vi "Config.vi"(8 "error in (no error)":errorcluster, 10 "Setting":variant, 11 "APS 7050":refnum<class "APS 7050.lvclass">) -> (0 "error out":errorcluster, 3 "APS 7050 out":refnum<class "APS 7050.lvclass">)   [LabVIEW 2025, in "Power Supply.lvlib" / "APS 7050.lvclass"]
uses:
  APS 7050.lvclass
  APS 7050.lvclass/APS 7050.ctl
  <instrlib>/APS-7000 Series/APS-7000 Series.lvlib
  PS Channel/Power Supply Channel.lvclass
  PS Channel configuration/Power Supply Channel configuration.lvclass
  Users/Public/Documents/Sandia National Labs/TSS Plugin/Abstract Engine.lvlibp/Plugin/Abstract/Abstract Instrument/Channel.ctl
  Users/Public/Documents/Sandia National Labs/TSS Plugin/Abstract Engine.lvlibp/Plugin/Abstract/Abstract Instrument/Abstract Instrument.lvclass
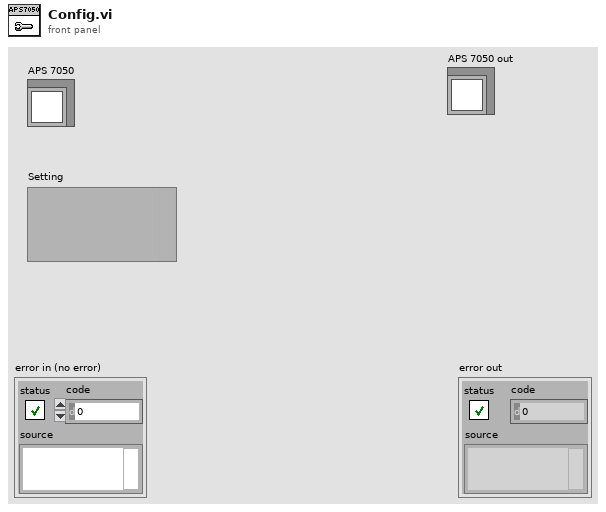
[diagram p1: front panel]
types:
  T1 = typedef "Abstract Engine.lvlibp/Abstract Instrument.lvclass/Channel.ctl" = cluster{"Alias":string, "DataType":enum16{"Anaolg Input", "Waveform"}, "Unit":enum16{"---", "V", "A", "Ohm", "Hz", "uF", "degC", "deg"}, "Upper limit":dbl, "Lower limit":dbl, "Measurement":variant}
  T2 = cluster{"Range":enum16{"R155", "R310", "R600", "AUTO"}, "FREQ":dbl, "ACV":dbl}
  T3 = typedef "Power Supply.lvlib/Power Supply Channel configuration.lvclass/PS Channel Setting.ctl" = cluster{"Driver":string, "Pin":string, "Test Voltage":string, "Voltage Low":dbl, "Voltage Norminal":dbl, "Voltage High":dbl, "PreTest Voltage":dbl, "PreTest Current":dbl, "Current Limit":dbl}
  T4 = typedef "Abstract Engine.lvlibp/Channel configuration.lvclass/Default Channel.ctl" = cluster{"Address":string, "SW Alias":string, "Enabled":bool, "Type":string, "Description":string}
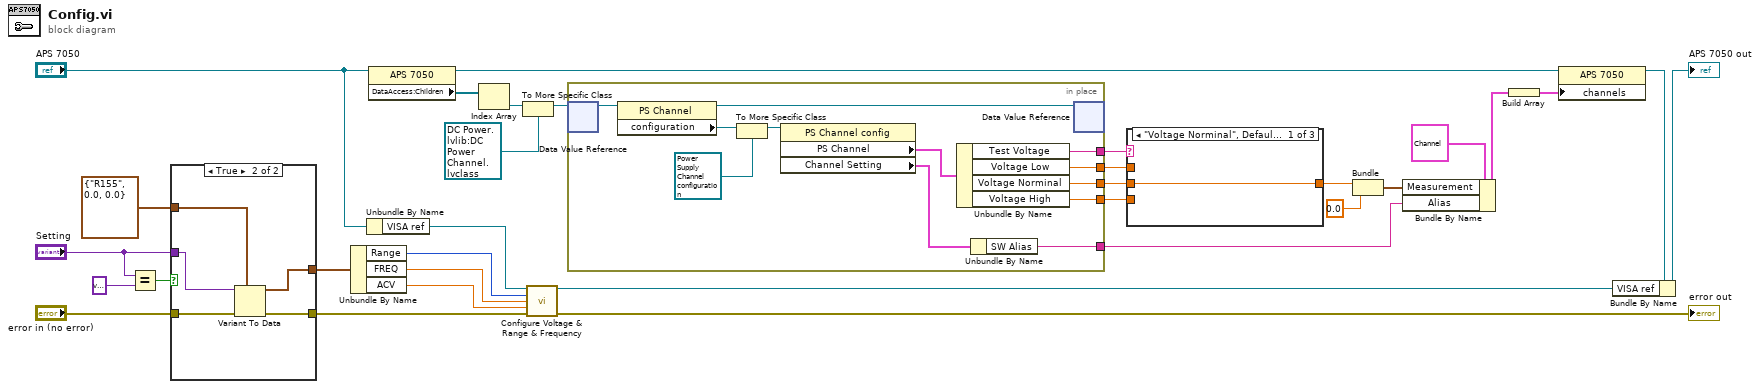
[diagram p0: block diagram]
diagram:
  n1 = Equal?(x="Setting", y=variant ("Setting")) -> (x = y?=w24:bool)
  n2 = case shown="True" w24 {
    tunnel: "Setting" -> [_ w37]
    tunnel: "error in (no error)" -> [w34 w39]
    tunnel: [w34 w38] -> w22
    tunnel: [w33 w36] -> w21
    tunnel: T2 {"Range"=enum."R155", "FREQ"=0.0, "ACV"=0.0} ("AC") -> [w33 w35]
    frame False {
    }
    frame True {
      n3 = Variant To Data(error in=w39, type=w35, Variant=w37) -> (data=w36:T2, error out=w38:errorcluster)
    }
  }
  n4 = Unbundle By Name(w21) -> ("Range"=w31:enum16{"R155", "R310", "R600", "AUTO"}, "FREQ"=w30:dbl, "ACV"=w29:dbl)
  n5 = Unbundle By Name("APS 7050") -> ("VISA ref"=w28:refnum<visa-resource-name>)
  n6 = property class="APS 7050"(reference="APS 7050") -> (reference out=w15:refnum<class "APS 7050.lvclass">, "DataAccess:Children"=w14:refnum<data-value>[])  [unwired: 1 in, 1 out]
  n7 = Index Array(array=w14) -> (element=w13:refnum<data-value>)  [unwired: 1 in]
  n8 = To More Specific Class(target class=refnum<data-value> refnum ("data value reference"), reference=w13) -> (specific class reference=w11:refnum<data-value>)  [unwired: 1 in, 1 out]
  n9 = call <instrlib>:"Configure Voltage & Range & Frequency.vi"("VISA in"=w28, "Range"=w31, "FREQ"=w30, "ACV"=w29, "error in"=w22) -> ("VISA out"=w25:refnum<visa-resource-name>, "error out"=→"error out":errorcluster)  [unwired: 2 in, 7 out]
  n10 = in-place {
    in-place-border: [w49] -> w6
    in-place-border: [w43] -> w10
    in-place-border: [w42] -> w9
    in-place-border: [w41] -> w8
    in-place-border: [w40] -> w7
    # "Initialize the front panel controls when loaded"
    n11 = in-place-dvr #1(w11) -> (w51:refnum<class "Power Supply Channel.lvclass">)  [unwired: 1 out]
    n12 = property class="PS Channel"(reference=w51) -> (reference out=w50:refnum<class "Power Supply Channel.lvclass">, "configuration"=w48:refnum<class "CEF_serializable configuration.lvclass">)  [unwired: 1 in, 1 out]
    n13 = To More Specific Class(target class=refnum<class "Power Supply Channel configuration.lvclass"> refnum ("DC Power.lvlib:DCPower Channel configuration.lvclass"), reference=w48) -> (specific class reference=w47:refnum<class "Power Supply Channel configuration.lvclass">)  [unwired: 1 in, 1 out]
    n14 = property class="PS Channel config"(reference=w47) -> ("PS Channel"=w45:T3, "Channel Setting"=w44:T4)  [unwired: 1 in, 2 out]
    n15 = Unbundle By Name(w45) -> ("Test Voltage"=w43:string, "Voltage Low"=w42:dbl, "Voltage Norminal"=w41:dbl, "Voltage High"=w40:dbl)
    n16 = Unbundle By Name(w44) -> ("SW Alias"=w49:string)
    n17 = in-place-dvr #1(w50) -> ()  [unwired: 2 out]
  }
  n18 = case shown="\"Voltage Norminal\", Default" w10 {
    tunnel: w9 -> [_ _ w54]
    tunnel: w8 -> [w52 _ _]
    tunnel: w7 -> [_ w53 _]
    tunnel: [w52 w53 w54] -> w5
    frame "Voltage Norminal", Default {
    }
    frame "Voltage High" {
    }
    frame "Voltage Low" {
    }
  }
  n19 = Bundle("Voltage Low"=w5, 0.0) -> (w4:cluster{"Voltage Low":dbl, dbl})  [unwired: 1 in]
  n20 = Bundle By Name(cluster=T1 {"Alias"="ch0", "DataType"=enum."Anaolg Input", "Unit"=enum."V", "Upper limit"=10.0, "Lower limit"=-10.0, "Measurement"=variant} ("Channel"), "Measurement"=w4, "Alias"=w6) -> (w16:T1)
  n21 = Build Array(w16) -> (w2:T1[])
  n22 = property class="APS 7050"(reference=w15, "channels"=w2) -> (reference out=w17:refnum<class "APS 7050.lvclass">)  [unwired: 1 in, 1 out]
  n23 = Bundle By Name(cluster=w17, "VISA ref"=w25) -> (→"APS 7050 out":refnum<class "APS 7050.lvclass">)
